vi "Configure Measurement (Spurious Emissions).vi"(0 "VISA resource name":refnum<visa-resource-name>, 1 "Enable Fast Spurious Measurement (Enable)":bool=TRUE, 5 "Measurement Type":u16(ring) items=["Examine", "Full"], 7 "Enable Auto Reference Level (T: Enable)":bool=TRUE, 9 "Manual Reference Level (10 dBm)":i32=10, 11 "error in (no error)":errorcluster) -> (4 "VISA resource name out":refnum<visa-resource-name>, 15 "error out":errorcluster)   [LabVIEW 2014, in "Agilent ESA PSA Series.lvlib"]
doc: "Sets up the spurious emissions measurement."
uses:
  Agilent ESA PSA Series.lvlib
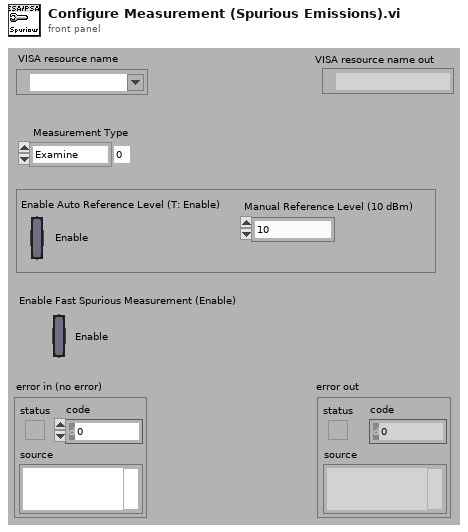
[diagram p1: front panel]
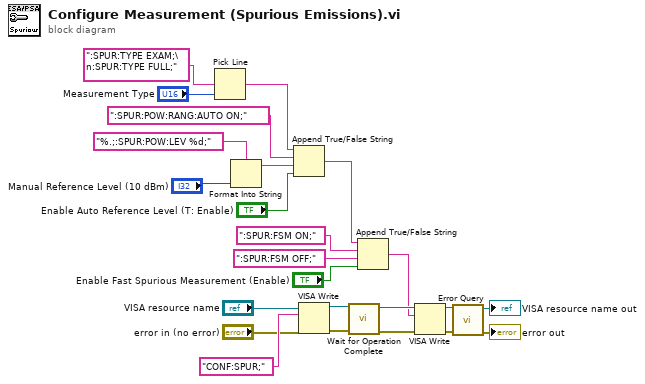
[diagram p0: block diagram]
diagram:
  n1 = Pick Line(multi-line string=":SPUR:TYPE EXAM;\n:SPUR:TYPE FULL;" ("format string"), line index="Measurement Type") -> (output string=w12:string)  [unwired: 1 in]
  n2 = Format Into String(format string="%.;:SPUR:POW:LEV %d;", "Manual Reference Level (10 dBm)") -> (resulting string=w21:string)  [unwired: 2 in, 1 out]
  n3 = Append True/False String(1:"Enable Auto Reference Level (T: Enable)", 2:w21, 3:":SPUR:POW:RANG:AUTO ON;" ("true string"), 4:w12) -> (0:w2:string)
  n4 = VISA Write(VISA resource name="VISA resource name", write buffer="CONF:SPUR;" ("string (\"\")"), error in (no error)="error in (no error)") -> (VISA resource name out=w6:refnum<visa-resource-name>, error out=w5:errorcluster)  [unwired: 1 out]
  n5 = call "Wait for Operation Complete.vi"("error in (no error)"=w5, "VISA resource name"=w6) -> ("error out"=w4:errorcluster, "VISA resource name out"=w3:refnum<visa-resource-name>)  [unwired: 8 in]
  n6 = Append True/False String(1:"Enable Fast Spurious Measurement (Enable)", 2:":SPUR:FSM OFF;" ("true string"), 3:":SPUR:FSM ON;" ("true string"), 4:w2) -> (0:w1:string)
  n7 = VISA Write(VISA resource name=w3, write buffer=w1, error in (no error)=w4) -> (VISA resource name out=w11:refnum<visa-resource-name>, error out=w10:errorcluster)  [unwired: 1 out]
  n8 = call "Error Query.vi"("error in (no error)"=w10, "VISA resource name"=w11) -> ("error out"=→"error out":errorcluster, "VISA resource name out"=→"VISA resource name out":refnum<visa-resource-name>)  [unwired: 6 in, 2 out]
